vi "Convert Relative to Absolute Coords.vi"(7 "Relative Movement Type":T1, 8 "error in (no error)":errorcluster, 9 "Relative Object Name":string, 10 "Y":i32, 11 "X":i32) -> (0 "error out":errorcluster, 2 "Abs Y":i32, 3 "Abs X":i32)   [LabVIEW 2020, in "MacroAssert.lvlib" / "Mouse Action.lvclass"]
uses:
  Mouse Action.lvclass
  Relative Movement Type.ctl
  SubVIs/Win Util/Win Util.lvlib
  MacroAssert.lvlib
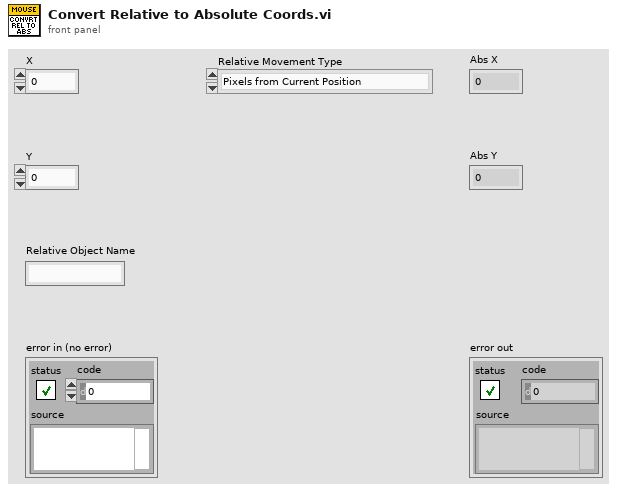
[diagram p1: front panel]
types:
  T1 = typedef "MacroAssert.lvlib/Mouse Action.lvclass/Relative Movement Type.ctl" = enum16{"Pixels from Current Position", "Pixels from Top-Left of Control", "Pixels from Top-Left of Window", "Percentage from Top-Left of Control", "Percentage from Top-Left of Window", "Percentage from Top-Left of Screen"}
  T2 = typedef "LVPositionTypeDef.ctl" = cluster{"Left":i32, "Top":i32}
  T3 = typedef "LVBoundsTypeDef.ctl" = cluster{"Width":u32, "Height":u32}
  T4 = typedef "LVPointTypeDef.ctl" = cluster{"Horizontal":i16, "Vertical":i16}
  T5 = typedef "MacroAssert.lvlib/Win Util.lvlib/Window Refnum.ctl" = u64
  T6 = cluster{"left":i16, "top":i16, "right":i16, "bottom":i16}
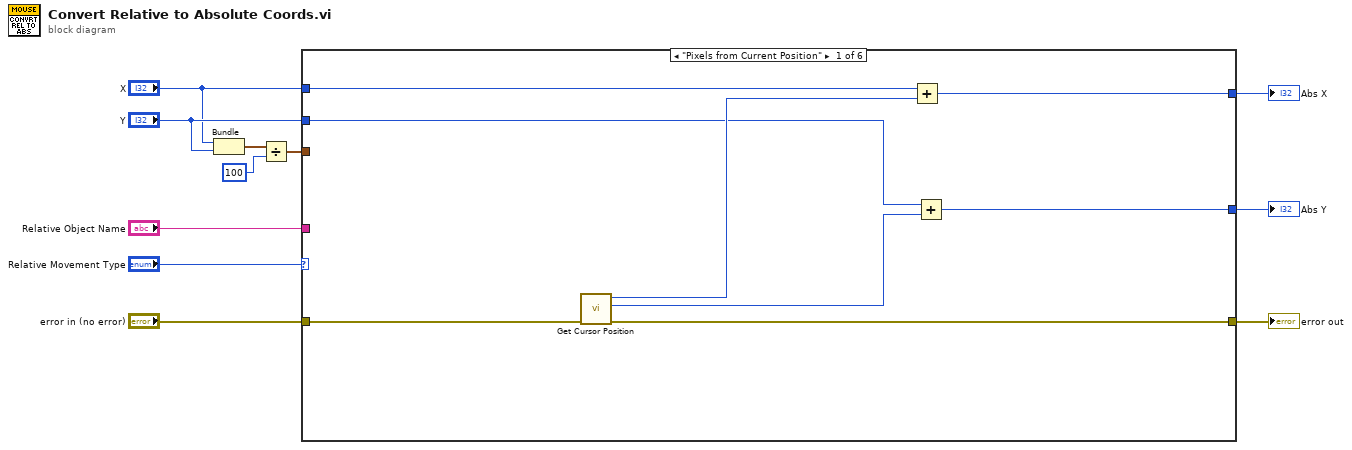
[diagram p0: block diagram]
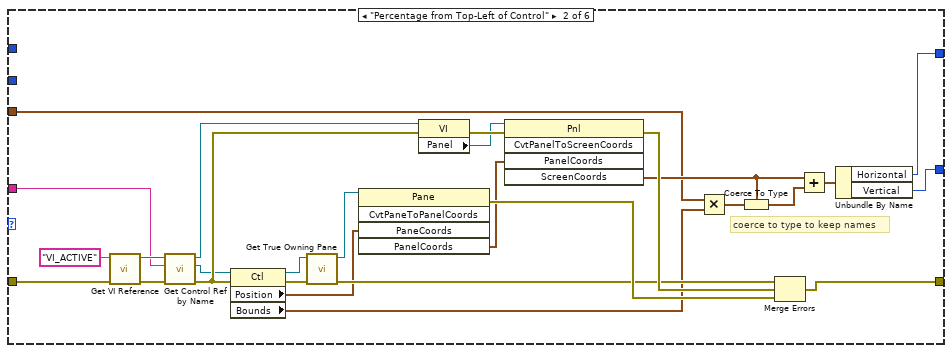
[diagram p2: hidden frame]
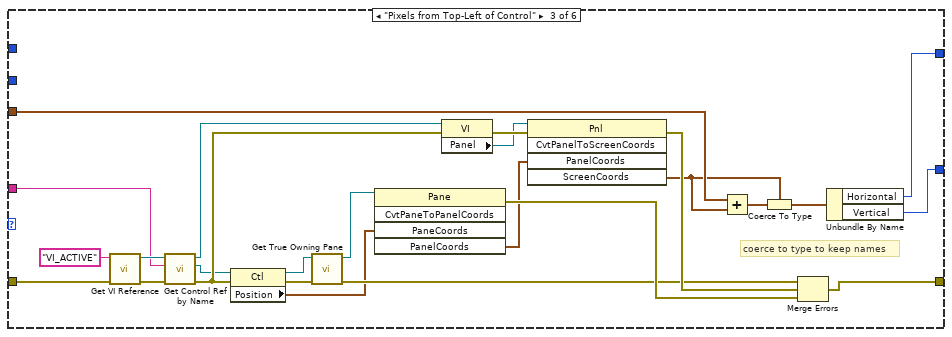
[diagram p3: hidden frame]
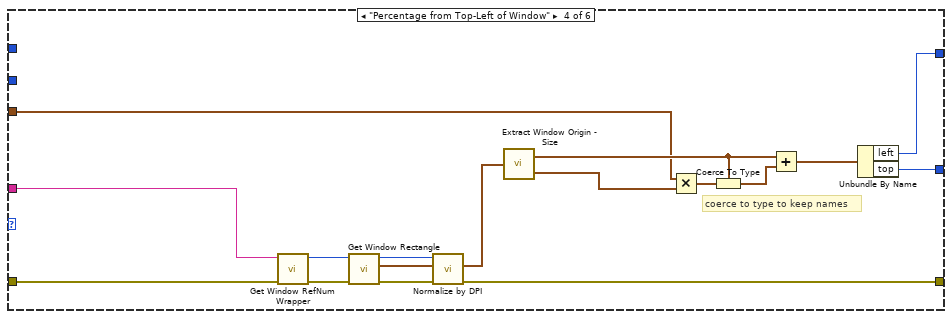
[diagram p4: hidden frame]
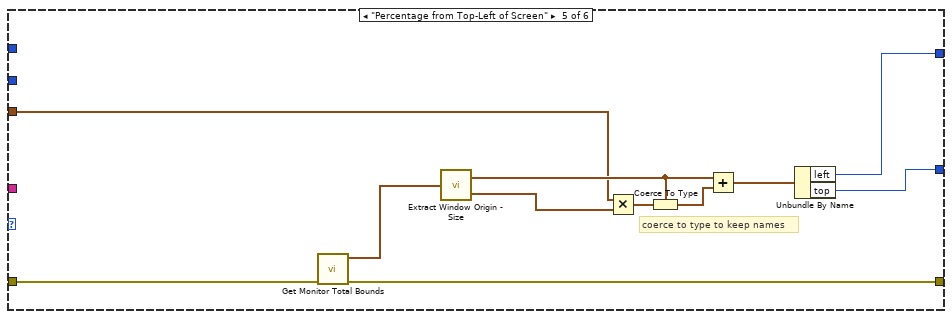
[diagram p5: hidden frame]
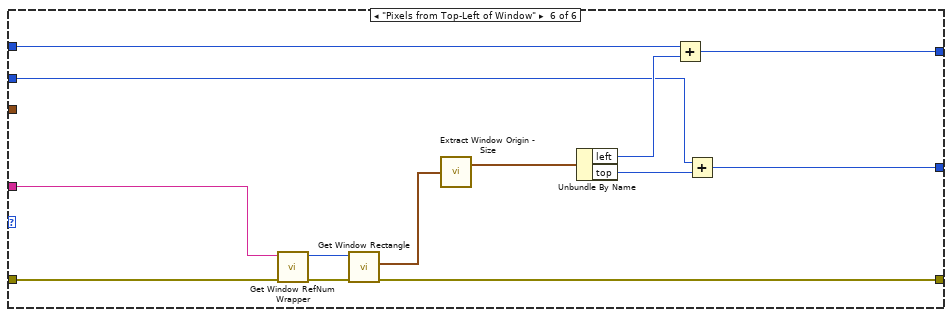
[diagram p6: hidden frame]
diagram:
  n1 = Bundle("X"="X", "Y"="Y") -> (w7:cluster{"X":i32, "Y":i32})  [unwired: 1 in]
  n2 = Divide(x=w7, y=100) -> (x/y=w5:cluster{"X":dbl, "Y":dbl})
  n3 = case shown="\"Pixels from Current Position\"" "Relative Movement Type" {
    tunnel: "error in (no error)" -> [w19 w42 w67 w87 w99 w111]
    tunnel: [w18 w39 w64 w85 w98 w110] -> w10
    tunnel: "Relative Object Name" -> [_ w31 w56 w83 _ w106]
    tunnel: [w15 w24 w53 w72 w93 w103] -> w4
    tunnel: w5 -> [_ w23 w52 w75 w91 _]
    tunnel: "Y" -> [w14 _ _ _ _ w101]
    tunnel: "X" -> [w17 _ _ _ _ w104]
    tunnel: [w12 w25 w54 w73 w94 w100] -> w1
    frame "Pixels from Current Position" {
      n4 = call "Get Cursor Position.vi"("error in (no error)"=w19) -> ("error out"=w18:errorcluster, "Y"=w13:i32, "X"=w16:i32)  [unwired: 8 in]
      n5 = Add(x=w17, y=w16) -> (x+y=w15:i32)
      n6 = Add(x=w14, y=w13) -> (x+y=w12:i32)
    }
    frame "Percentage from Top-Left of Control" {
      # "coerce to type to keep names"
      n7 = call "Get VI Reference.vi"("error in (no error)"=w42, "VI Name"="VI_ACTIVE") -> ("error out"=w41:errorcluster, "VI Ref"=w37:refnum<vi>)  [unwired: 8 in]
      n8 = call "Get Control Ref by Name.vi"("error in (no error)"=w41, "Name"=w31, "VI Ref"=w37) -> ("error out"=w44:errorcluster, "Ctl Ref"=w36:refnum<vi>, "VI Ref out"=w35:refnum<vi>)  [unwired: 6 in]
      n9 = property class="Ctl"(reference=w36, error in=w44) -> (reference out=w33:refnum<vi>, error out=w40:errorcluster, "Position"=w21:T2, "Bounds"=w30:T3)
      n10 = call "Get True Owning Pane.vi"("error in (no error)"=w40, "Ctl Ref"=w33) -> ("error out"=w38:errorcluster, "Owning Pane"=w32:refnum<vi>)  [unwired: 8 in]
      n11 = invoke class="Pane" method="CvtPaneToPanelCoords"(reference=w32, "PaneCoords"=w21) -> (error out=w45:errorcluster, "PanelCoords"=w22:T4)  [unwired: 3 in, 3 out]
      n12 = property class="VI"(reference=w35, error in=w44) -> (error out=w43:errorcluster, "Panel"=w34:refnum<vi>)  [unwired: 1 out]
      n13 = invoke class="Pnl" method="CvtPanelToScreenCoords"(reference=w34, error in=w43, "PanelCoords"=w22) -> (error out=w46:errorcluster, "ScreenCoords"=w27:T4)  [unwired: 2 in, 3 out]
      n14 = Multiply(x=w23, y=w30) -> (x*y=w29:cluster{dbl, dbl})
      n15 = Coerce To Type(0:w29, 1:w27) -> (2:w28:T4)
      n16 = Merge Errors(w38, w46, w45) -> (w39:errorcluster)
      n17 = Add(x=w27, y=w28) -> (x+y=w26:T4)
      n18 = Unbundle By Name(w26) -> ("Horizontal"=w24:i16, "Vertical"=w25:i16)
    }
    frame "Pixels from Top-Left of Control" {
      # "coerce to type to keep names"
      n19 = call "Get VI Reference.vi"("error in (no error)"=w67, "VI Name"="VI_ACTIVE") -> ("error out"=w66:errorcluster, "VI Ref"=w62:refnum<vi>)  [unwired: 8 in]
      n20 = call "Get Control Ref by Name.vi"("error in (no error)"=w66, "Name"=w56, "VI Ref"=w62) -> ("error out"=w69:errorcluster, "Ctl Ref"=w61:refnum<vi>, "VI Ref out"=w60:refnum<vi>)  [unwired: 6 in]
      n21 = property class="Ctl"(reference=w61, error in=w69) -> (reference out=w58:refnum<vi>, error out=w65:errorcluster, "Position"=w50:T2)
      n22 = call "Get True Owning Pane.vi"("error in (no error)"=w65, "Ctl Ref"=w58) -> ("error out"=w63:errorcluster, "Owning Pane"=w57:refnum<vi>)  [unwired: 8 in]
      n23 = invoke class="Pane" method="CvtPaneToPanelCoords"(reference=w57, "PaneCoords"=w50) -> (error out=w70:errorcluster, "PanelCoords"=w51:T4)  [unwired: 3 in, 3 out]
      n24 = property class="VI"(reference=w60, error in=w69) -> (error out=w68:errorcluster, "Panel"=w59:refnum<vi>)  [unwired: 1 out]
      n25 = invoke class="Pnl" method="CvtPanelToScreenCoords"(reference=w59, error in=w68, "PanelCoords"=w51) -> (error out=w71:errorcluster, "ScreenCoords"=w49:T4)  [unwired: 2 in, 3 out]
      n26 = Add(x=w52, y=w49) -> (x+y=w55:cluster{dbl, dbl})
      n27 = Coerce To Type(0:w55, 1:w49) -> (2:w48:T4)
      n28 = Merge Errors(w63, w71, w70) -> (w64:errorcluster)
      n29 = Unbundle By Name(w48) -> ("Horizontal"=w53:i16, "Vertical"=w54:i16)
    }
    frame "Percentage from Top-Left of Window" {
      # "coerce to type to keep names"
      n30 = call "Get Window RefNum Wrapper.vi"("error in (no error)"=w87, "Window Name"=w83) -> ("error out"=w88:errorcluster, "window refnum"=w84:T5)  [unwired: 8 in]
      n31 = call "Get Window Rectangle.vi"("error in (no error)"=w88, "window refnum (NaWR)"=w84) -> ("error out"=w86:errorcluster, "window rect"=w81:T6, "window refnum out"=w82:T5)  [unwired: 7 in]
      n32 = call "Normalize by DPI.vi"("error in (no error)"=w86, "window rect"=w81, "window refnum (NaWR)"=w82) -> ("error out"=w85:errorcluster, "normalized window rect"=w74:T6)  [unwired: 6 in, 1 out]
      n33 = call "Extract Window Origin - Size.vi"("window rect"=w74) -> ("window origin"=w77:cluster{"left":i16, "top":i16}, "window size"=w76:cluster{"Width":i16, "Height":i16})
      n34 = Multiply(x=w75, y=w76) -> (x*y=w80:cluster{dbl, dbl})
      n35 = Coerce To Type(0:w80, 1:w77) -> (2:w79:cluster{"left":i16, "top":i16})
      n36 = Add(x=w77, y=w79) -> (x+y=w78:cluster{"left":i16, "top":i16})
      n37 = Unbundle By Name(w78) -> ("left"=w72:i16, "top"=w73:i16)
    }
    frame "Percentage from Top-Left of Screen" {
      # "coerce to type to keep names"
      n38 = call "Get Monitor Total Bounds.vi"("error in (no error)"=w99) -> ("error out"=w98:errorcluster, "window rect"=w90:T6)  [unwired: 9 in]
      n39 = call "Extract Window Origin - Size.vi"("window rect"=w90) -> ("window origin"=w92:cluster{"left":i16, "top":i16}, "window size"=w89:cluster{"Width":i16, "Height":i16})
      n40 = Multiply(x=w91, y=w89) -> (x*y=w97:cluster{dbl, dbl})
      n41 = Coerce To Type(0:w97, 1:w92) -> (2:w96:cluster{"left":i16, "top":i16})
      n42 = Add(x=w92, y=w96) -> (x+y=w95:cluster{"left":i16, "top":i16})
      n43 = Unbundle By Name(w95) -> ("left"=w93:i16, "top"=w94:i16)
    }
    frame "Pixels from Top-Left of Window" {
      n44 = call "Get Window RefNum Wrapper.vi"("error in (no error)"=w111, "Window Name"=w106) -> ("error out"=w112:errorcluster, "window refnum"=w109:T5)  [unwired: 8 in]
      n45 = call "Get Window Rectangle.vi"("error in (no error)"=w112, "window refnum (NaWR)"=w109) -> ("error out"=w110:errorcluster, "window rect"=w108:T6)  [unwired: 7 in, 1 out]
      n46 = call "Extract Window Origin - Size.vi"("window rect"=w108) -> ("window origin"=w107:cluster{"left":i16, "top":i16})  [unwired: 1 out]
      n47 = Unbundle By Name(w107) -> ("left"=w105:i16, "top"=w102:i16)
      n48 = Add(x=w104, y=w105) -> (x+y=w103:i32)
      n49 = Add(x=w101, y=w102) -> (x+y=w100:i32)
    }
  }
  "error out" <- w10
  "Abs X" <- w4
  "Abs Y" <- w1
